vi "RTS Read Point File.vi"(8 "Error In":errorcluster, 11 "Path":path) -> (0 "Error Out":errorcluster, 2 "Array 2":string[](array[string]), 3 "Point File":T1[](array[typedef]))   [LabVIEW 2016]
uses:
  Type Definitions/RTS Point File.ctl
  <vilib>/Utility/file.llb/Read Delimited Spreadsheet (string).vi
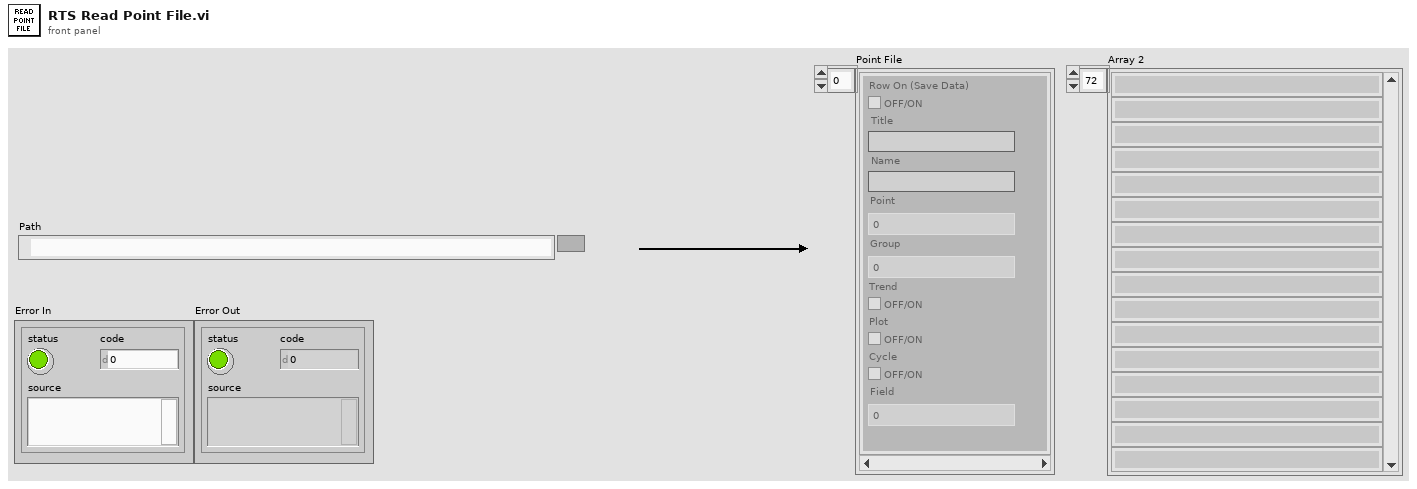
[diagram p1: front panel]
types:
  T1 = typedef "RTS Point File.ctl" = cluster{"Title":string, "Name":string, "Point":u8, "Plot":bool, "Trend":bool, "Cycle":bool, "Field":u8, "Row On (Save Data)":bool, "Group":u8}
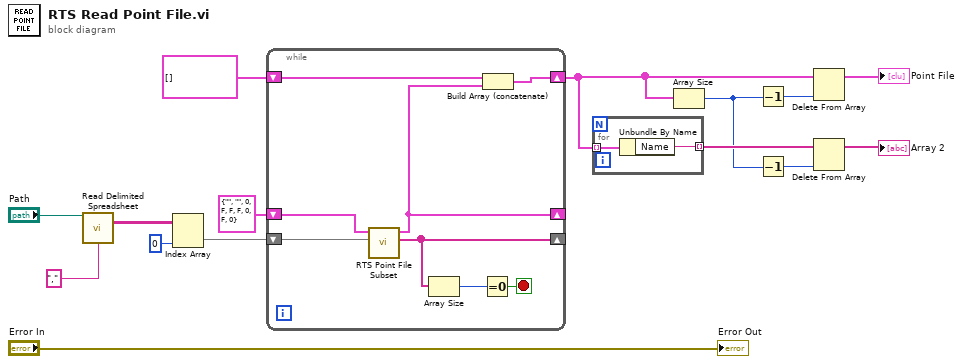
[diagram p0: block diagram]
diagram:
  n1 = call-poly <vilib>:"Read Delimited Spreadsheet.vi"("file path (dialog if empty)"="Path", "delimiter (\\t)"="," ("delimiter (\\t)")) -> ("all rows"=w14:string[][])  [unwired: 8 in, 5 out]
  n2 = Index Array(array=w14, index (col)=0 ("disabled index (col)")) -> (element=w8:string[])  [unwired: 1 in]
  n3 = while {
    shift-right: [w21] -> _
    shift-left: w8 -> [w23]
    shift-right: [w18] -> _
    shift-left: T1 {"Title"="", "Name"="", "Point"=0, "Plot"=FALSE, "Trend"=FALSE, "Cycle"=FALSE, "Field"=0, "Row On (Save Data)"=FALSE, "Group"=0} ("Point File Input") -> [w22]
    shift-right: [w19] -> w7
    shift-left: T1[] [] -> [w20]
    stop <- w17 stop-if-true
    n4 = call "RTS Point File Subset.vi"("Data Input"=w23, "Point File Input"=w22) -> ("Next Subset"=w21:string[], "Point File Output"=w18:T1)  [unwired: 7 in, 1 out]
    n5 = Array Size(array=w21) -> (size(s)=w16:i32)
    n6 = Equal To 0?(x=w16) -> (x = 0?=w17:bool)
    n7 = Build Array (concatenate)(w20, w18) -> (w19:T1[])
  }
  n8 = for {
    tunnel: w7 -> [w25] mode=indexing
    tunnel: [w24] -> w3 mode=indexing
    n9 = Unbundle By Name(w25) -> ("Name"=w24:string)
  }
  n10 = Array Size(array=w7) -> (size(s)=w1:i32)
  n11 = Decrement(x=w1) -> (x-1=w6:i32)
  n12 = Decrement(x=w1) -> (x-1=w4:i32)
  n13 = Delete From Array(array=w7, index=w6) -> (array with subset deleted=→"Point File":T1[])  [unwired: 1 in, 1 out]
  n14 = Delete From Array(array=w3, index=w4) -> (array with subset deleted=→"Array 2":string[])  [unwired: 1 in, 1 out]
  "Error Out" <- "Error In"
